vi "CRYPrefix Curve Name.vi"(0 "Type In":string="NameChange", 5 "Curves In":T2 {"Z data" items=["dB", "Lin"]; "X data" items=["dB", "Lin"]; "Y data" items=["dB", "Lin"]; "Z dB ref" format="%.1f"; "Z axis" items=["Log", "Lin"]; "X dB ref" format="%.1f"; "X axis" items=["Log", "Lin"]; "Y axis" items=["Log", "Lin"]; "Y dB ref" format="%.1f"; "Curve"."z" format="%.2f"; "Curve"."y" format="%.2f"; "Curve"."x" format="%.2f"}, 7 "Values In":T2 {"Z data" items=["dB", "Lin"]; "X data" items=["dB", "Lin"]; "Y data" items=["dB", "Lin"]; "Z dB ref" format="%.1f"; "Z axis" items=["Log", "Lin"]; "X dB ref" format="%.1f"; "X axis" items=["Log", "Lin"]; "Y axis" items=["Log", "Lin"]; "Y dB ref" format="%.1f"; "Curve"."z" format="%.2f"; "Curve"."y" format="%.2f"; "Curve"."x" format="%.2f"}, 9 "Results In":T4 {"Margin" format="%.2f"}, 11 "Waves In":T6 {"Y dB ref" format="%.1f"; "Y axis" items=["Log", "Lin"]; "Y data" items=["dB", "Lin"]; "X data" items=["dB", "Lin"]}, 12 "Repeat State Array In":T1(array[cluster])) -> (6 "Curves Out":T2 {"Z data" items=["dB", "Lin"]; "X data" items=["dB", "Lin"]; "Y data" items=["dB", "Lin"]; "Z dB ref" format="%.1f"; "Z axis" items=["Log", "Lin"]; "X dB ref" format="%.1f"; "X axis" items=["Log", "Lin"]; "Y axis" items=["Log", "Lin"]; "Y dB ref" format="%.1f"; "Curve"."z" format="%.2f"; "Curve"."y" format="%.2f"; "Curve"."x" format="%.2f"}, 8 "Values Out":T2 {"Z data" items=["dB", "Lin"]; "X data" items=["dB", "Lin"]; "Y data" items=["dB", "Lin"]; "Z dB ref" format="%.1f"; "Z axis" items=["Log", "Lin"]; "X dB ref" format="%.1f"; "X axis" items=["Log", "Lin"]; "Y axis" items=["Log", "Lin"]; "Y dB ref" format="%.1f"; "Curve"."z" format="%.2f"; "Curve"."y" format="%.2f"; "Curve"."x" format="%.2f"}, 10 "Results Out":T4 {"Margin" format="%.2f"}, 15 "Waves Out":T6 {"Y dB ref" format="%.1f"; "Y axis" items=["Log", "Lin"]; "Y data" items=["dB", "Lin"]; "X data" items=["dB", "Lin"]})   [LabVIEW 2013]
uses:
  Typedef Control/CRYData Cluster Array.ctl
  Typedef Control/CRYData Cluster.ctl
  Typedef Control/CRYResult Cluster Array.ctl
  Typedef Control/CRYResult Cluster.ctl
  Typedef Control/CRYWaveform Cluster Array.ctl
  Typedef Control/CRYWaveform Cluster.ctl
  CRYProject Run Control Global.vi
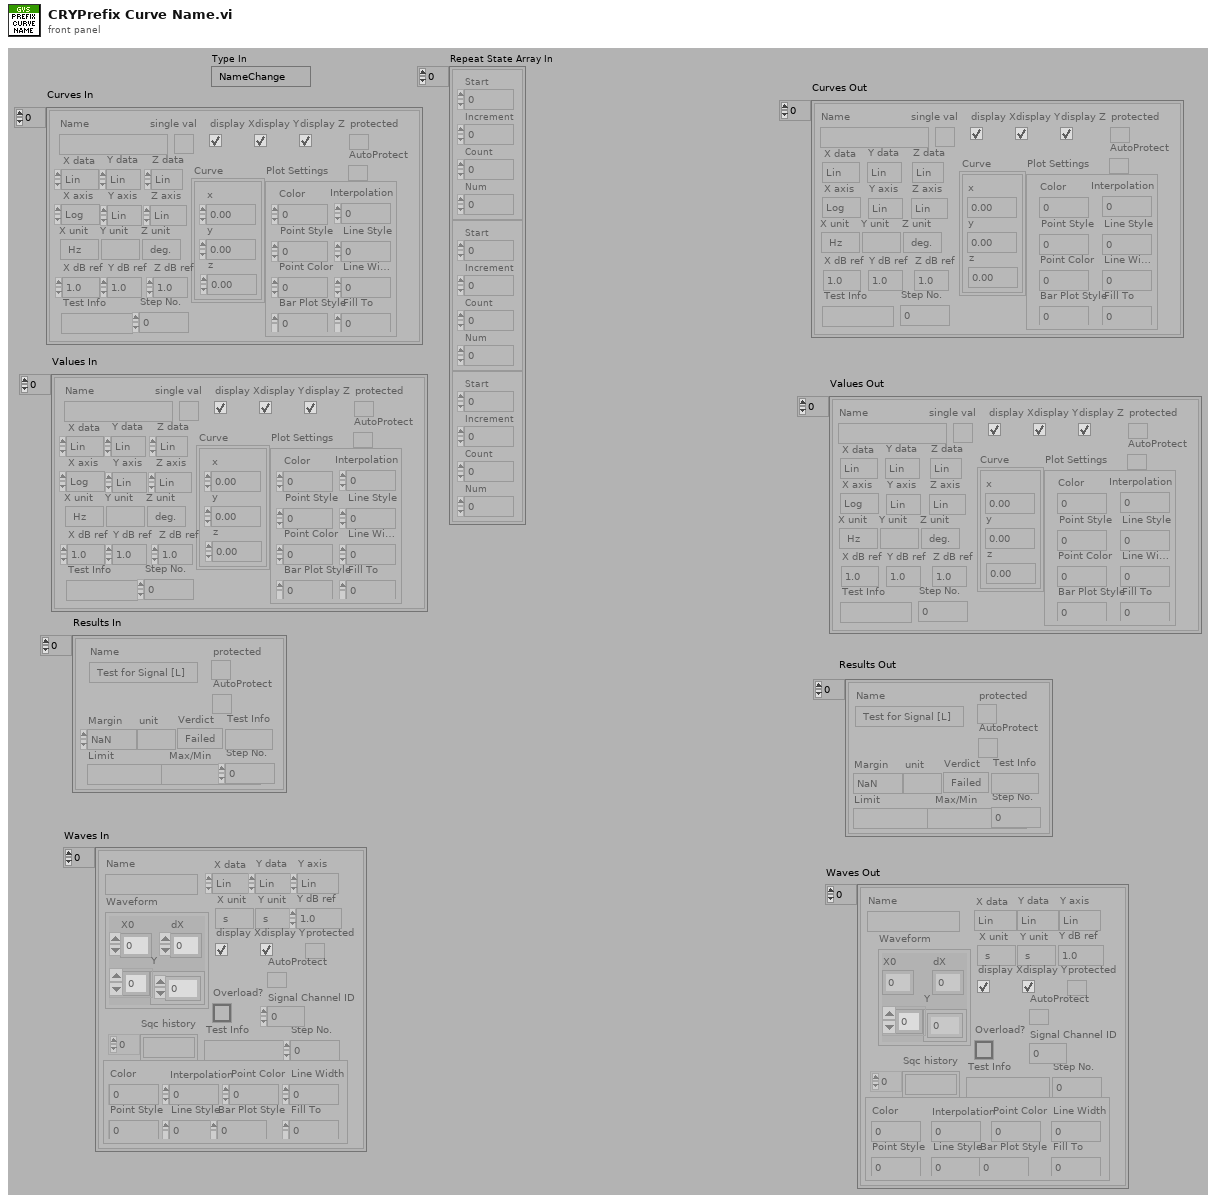
[diagram p1: front panel]
types:
  T1 = cluster{"Start":dbl, "Increment":dbl, "Count":i32, "Num":i32}[]
  T2 = typedef "CRYData Cluster Array.ctl" = T3[]
  T3 = typedef "CRYData Cluster.ctl" = cluster{"Name":string, "Curve":cluster{"x":dbl, "y":dbl, "z":dbl}[], "X data":u16, "Y data":u16, "Z data":u16, "X axis":u16, "Y axis":u16, "Z axis":u16, "X unit":string, "Y unit":string, "Z unit":string, "X dB ref":dbl, "Y dB ref":dbl, "Z dB ref":dbl, "single val":bool, "protected":bool, "display X":bool, "display Y":bool, "display Z":bool, "Test Info":string, "Step No.":i32, "Plot Settings":cluster{"Color":u32, "Interpolation":u8, "Point Style":u8, "Line Style":u8, "Point Color":u32, "Line Width":u8, "Bar Plot Style":u8, "Fill To":i16}, "AutoProtect":bool}
  T4 = typedef "CRYResult Cluster Array.ctl" = T5[]
  T5 = typedef "CRYResult Cluster.ctl" = cluster{"Name":string, "Margin":dbl, "unit":string, "Verdict":bool, "Limit":string, "Max/Min":string, "protected":bool, "Step No.":i32, "Test Info":string, "AutoProtect":bool}
  T6 = typedef "CRYWaveform Cluster Array.ctl" = T7[]
  T7 = typedef "CRYWaveform Cluster.ctl" = cluster{"Waveform":cluster{"X0":dbl, "dX":dbl, "Y":sgl[]}, "X data":u16, "Y data":u16, "Y axis":u16, "X unit":string, "Y unit":string, "Y dB ref":dbl, "display Y":bool, "display X":bool, "Overload?":bool, "Test Info":string, "Step No.":i32, "Name":string, "protected":bool, "Sqc history":string[], "Signal Channel ID":i32, "Plot Settings":cluster{"Color":u32, "Interpolation":u8, "Point Style":u8, "Line Style":u8, "Point Color":u32, "Line Width":u8, "Bar Plot Style":u8, "Fill To":i16}, "AutoProtect":bool}
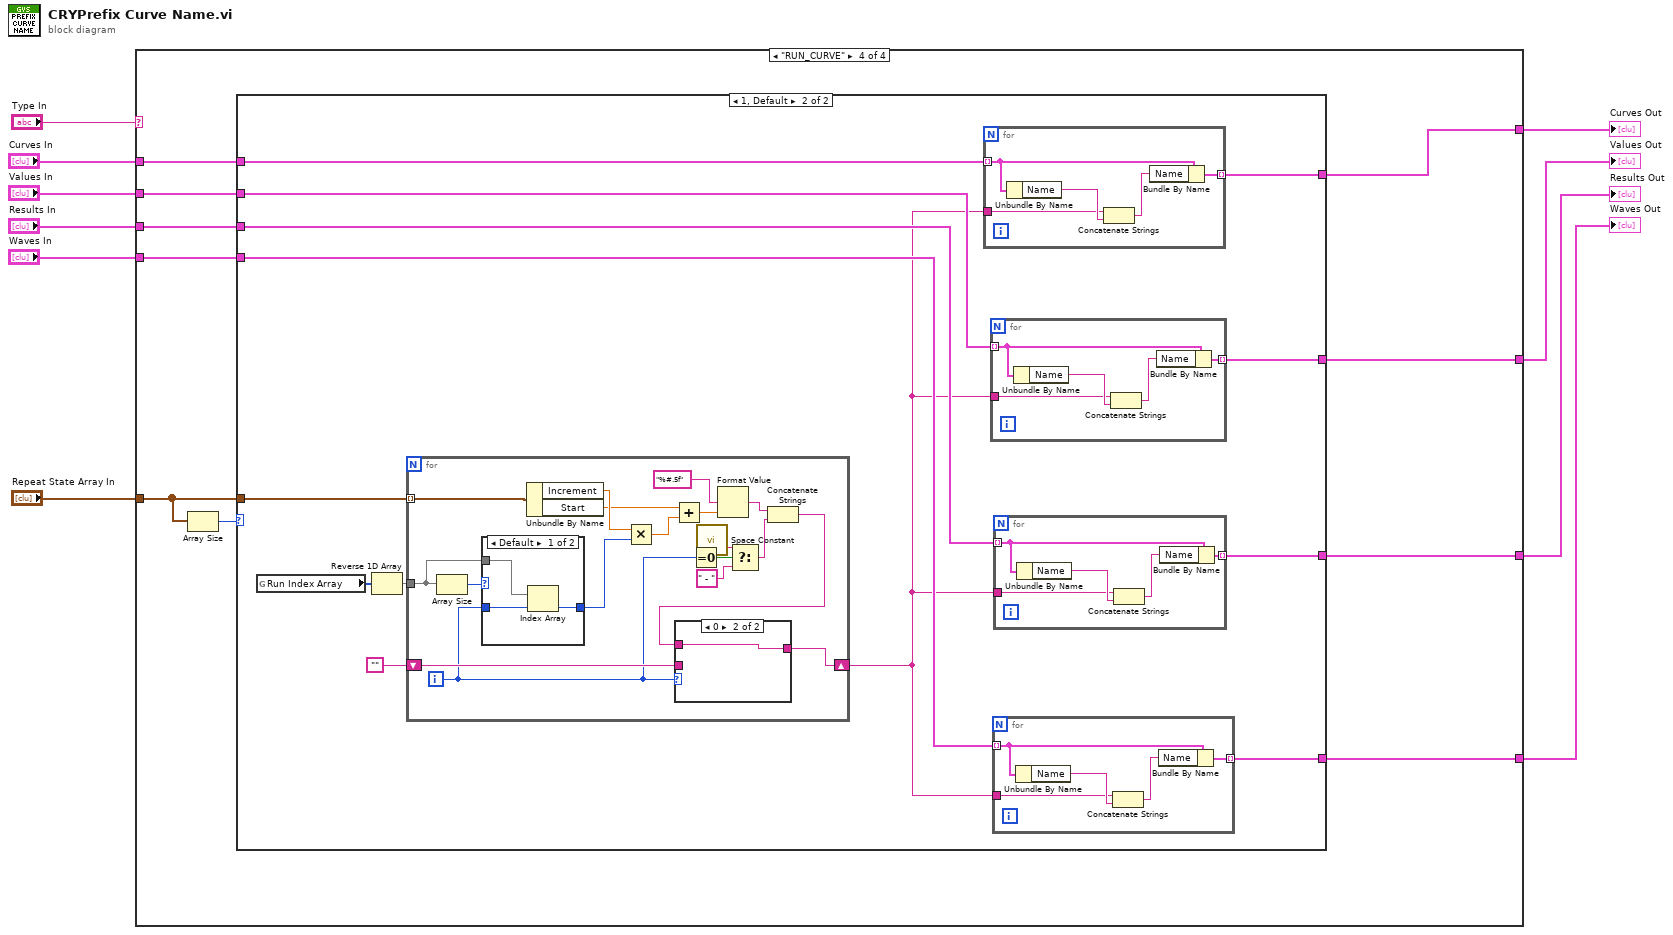
[diagram p0: block diagram]
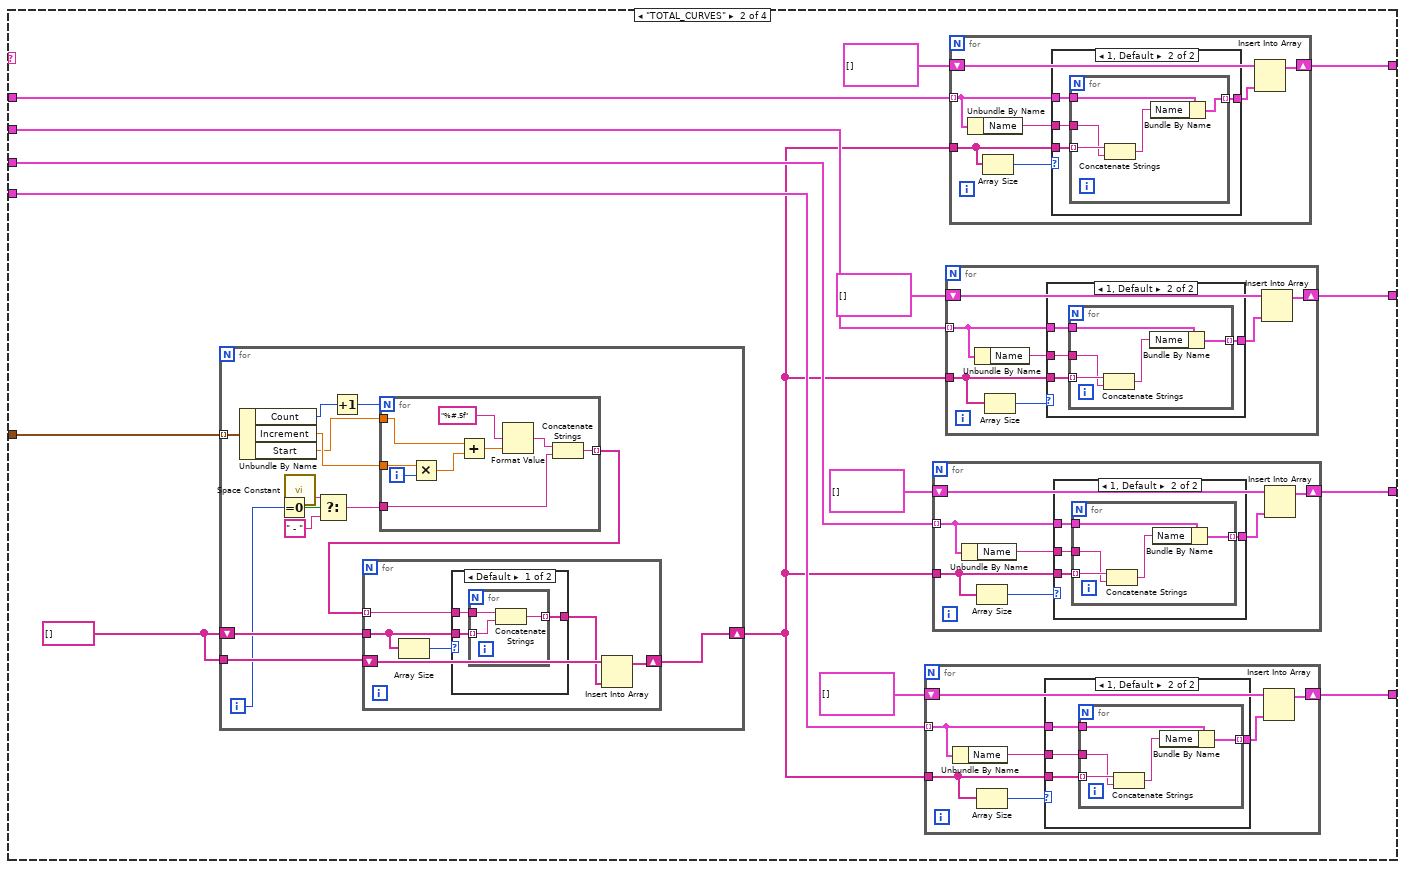
[diagram p3: hidden frame]
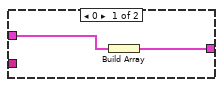
[diagram p4: hidden frame]
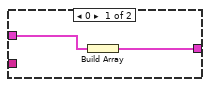
[diagram p5: hidden frame]
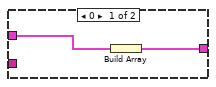
[diagram p6: hidden frame]
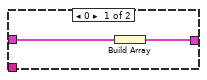
[diagram p7: hidden frame]
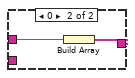
[diagram p8: hidden frame]
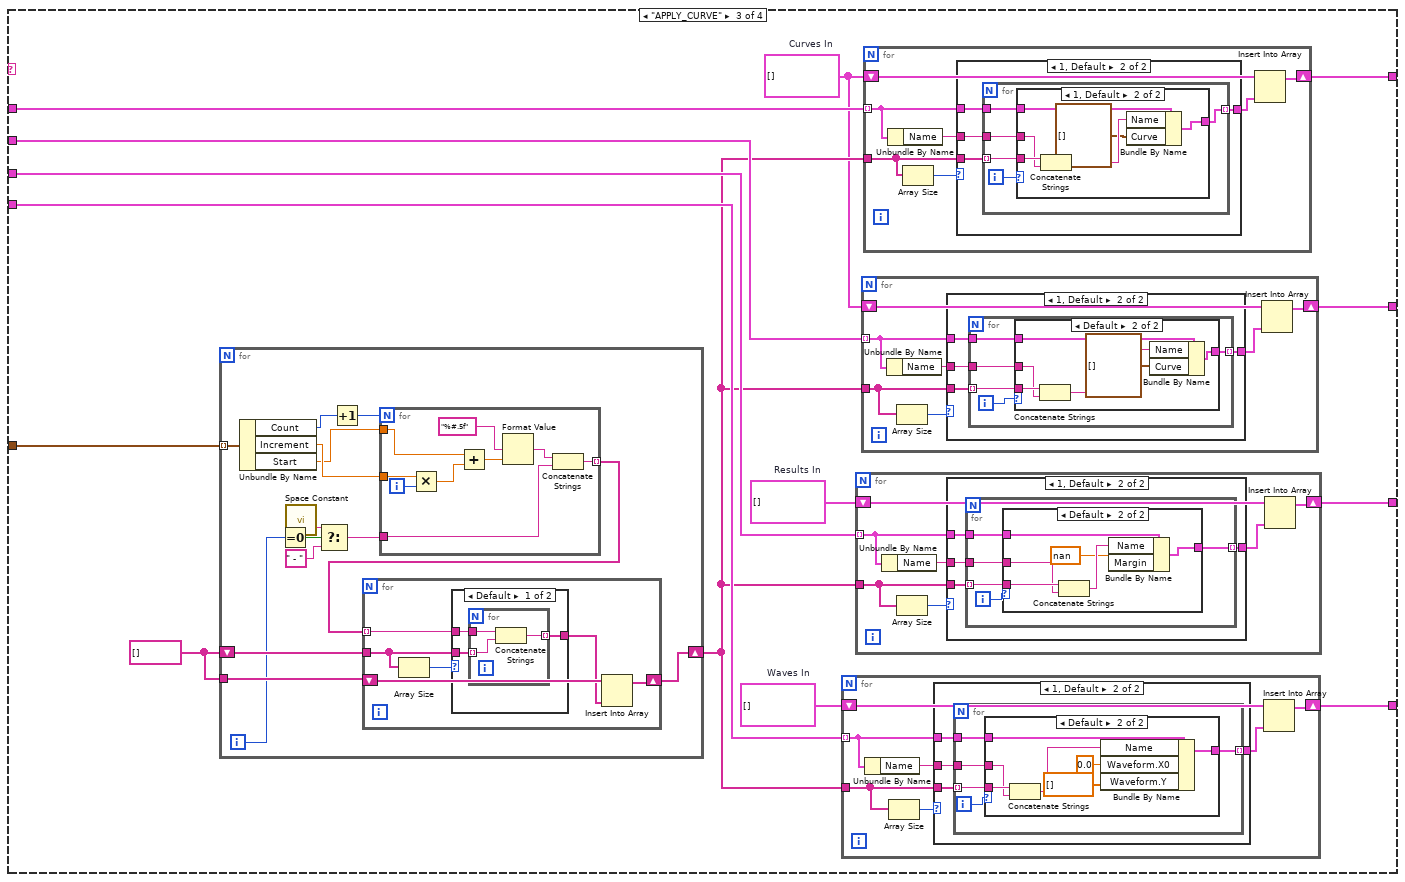
[diagram p9: hidden frame]
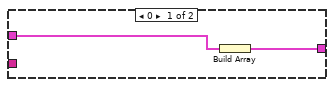
[diagram p10: hidden frame]
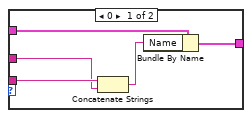
[diagram p11: hidden frame]
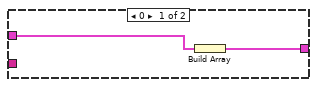
[diagram p12: hidden frame]
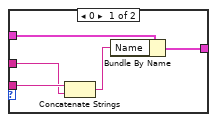
[diagram p13: hidden frame]
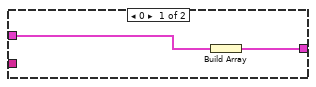
[diagram p14: hidden frame]
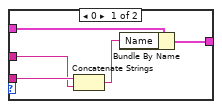
[diagram p15: hidden frame]
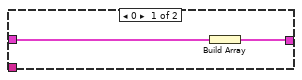
[diagram p16: hidden frame]
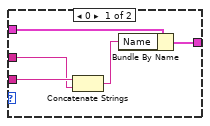
[diagram p17: hidden frame]
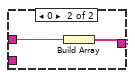
[diagram p18: hidden frame]
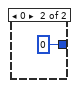
[diagram p20: hidden frame]
diagram:
  n1 = case shown="\"RUN_CURVE\"" "Type In" {
    tunnel: "Curves In" -> [_ w23 w146 w312]
    tunnel: "Repeat State Array In" -> [_ w24 w147 w308]
    tunnel: "Values In" -> [_ w22 w145 w311]
    tunnel: "Results In" -> [_ w20 w144 w310]
    tunnel: "Waves In" -> [_ w19 w143 w309]
    tunnel: [_ w15 w139 w307] -> w4
    tunnel: [_ w14 w138 w306] -> w3
    tunnel: [_ w13 w137 w305] -> w2
    tunnel: [_ w12 w136 w304] -> w1
    frame Default {
    }
    frame "TOTAL_CURVES" {
      w25 = string[] []
      n2 = for {
        tunnel: w24 -> [w111] mode=indexing
        shift-right: [w106] -> w18
        shift-left: w25 -> [w108]
        tunnel: w25 -> [w107]
        i -> [w99]
        n3 = Unbundle By Name(w111) -> ("Count"=w105:i32, "Increment"=w110:dbl, "Start"=w104:dbl)
        n4 = Equal To 0?(x=w99) -> (x = 0?=w102:bool)
        n5 = call <vilib>:"Space Constant.vi"() -> ("String"=w100:string)
        n6 = Select(t=w100, s=w102, f=" - " ("string")) -> (s? t:f=w98:string)
        n7 = Increment(x=w105) -> (x+1=w103:i32)
        n8 = for {
          N: w103 -> [_]
          tunnel: w104 -> [w134]
          tunnel: w110 -> [w133]
          tunnel: [w130] -> w109 mode=indexing
          tunnel: w98 -> [w126]
          i -> [w132]
          n9 = Multiply(x=w133, y=w132) -> (x*y=w131:dbl)
          n10 = Add(x=w134, y=w131) -> (x+y=w128:dbl)
          n11 = Format Value(format string="%#.5f", value (0)=w128) -> (output string=w127:string)  [unwired: 1 in]
          n12 = Concatenate Strings(w127, w126) -> (w130:string)
        }
        n13 = for {
          tunnel: w109 -> [w117] mode=indexing
          tunnel: w108 -> [w113]
          shift-right: [w115] -> w106
          shift-left: w107 -> [w116]
          n14 = Array Size(array=w113) -> (size(s)=w112:i32)
          n15 = case shown="Default" w112 {
            tunnel: w117 -> [w120 w125]
            tunnel: w113 -> [w119 _]
            tunnel: [w118 w124] -> w114
            frame Default {
              n16 = for {
                tunnel: w120 -> [w123]
                tunnel: w119 -> [w122] mode=indexing
                tunnel: [w121] -> w118 mode=indexing
                n17 = Concatenate Strings(w123, w122) -> (w121:string)
              }
            }
            frame 0 {
              n18 = Build Array(w125) -> (w124:string[])
            }
          }
          n19 = Insert Into Array(array=w116, new element=w114) -> (w115:string[])  [unwired: 1 in]
        }
      }
      n20 = for {
        tunnel: w19 -> [w31] mode=indexing
        tunnel: w18 -> [w27]
        shift-right: [w28] -> w12
        shift-left: T6 [] ("Waves In") -> [w30]
        n21 = Unbundle By Name(w31) -> ("Name"=w32:string)
        n22 = Array Size(array=w27) -> (size(s)=w26:i32)
        n23 = case shown="1, Default" w26 {
          tunnel: w32 -> [_ w38]
          tunnel: w31 -> [w34 w37]
          tunnel: [w33 w36] -> w29
          tunnel: w27 -> [_ w35]
          frame 0 {
            n24 = Build Array(w34) -> (w33:T7[])
          }
          frame 1, Default {
            n25 = for {
              tunnel: w38 -> [w42]
              tunnel: w35 -> [w43] mode=indexing
              tunnel: w37 -> [w41]
              tunnel: [w39] -> w36 mode=indexing
              n26 = Concatenate Strings(w43, w42) -> (w40:string)
              n27 = Bundle By Name(cluster=w41, "Name"=w40) -> (w39:T7)
            }
          }
        }
        n28 = Insert Into Array(array=w30, new element=w29) -> (w28:T6)  [unwired: 1 in]
      }
      n29 = for {
        tunnel: w20 -> [w49] mode=indexing
        tunnel: w18 -> [w45]
        shift-right: [w46] -> w13
        shift-left: T4 [] ("Results In") -> [w48]
        n30 = Unbundle By Name(w49) -> ("Name"=w50:string)
        n31 = Array Size(array=w45) -> (size(s)=w44:i32)
        n32 = case shown="1, Default" w44 {
          tunnel: w50 -> [_ w56]
          tunnel: w45 -> [_ w55]
          tunnel: w49 -> [w52 w54]
          tunnel: [w51 w53] -> w47
          frame 0 {
            n33 = Build Array(w52) -> (w51:T5[])
          }
          frame 1, Default {
            n34 = for {
              tunnel: w56 -> [w60]
              tunnel: w55 -> [w61] mode=indexing
              tunnel: w54 -> [w59]
              tunnel: [w57] -> w53 mode=indexing
              n35 = Concatenate Strings(w61, w60) -> (w58:string)
              n36 = Bundle By Name(cluster=w59, "Name"=w58) -> (w57:T5)
            }
          }
        }
        n37 = Insert Into Array(array=w48, new element=w47) -> (w46:T4)  [unwired: 1 in]
      }
      n38 = for {
        tunnel: w22 -> [w67] mode=indexing
        tunnel: w18 -> [w63]
        shift-right: [w64] -> w14
        shift-left: T2 [] ("Values In") -> [w66]
        n39 = Unbundle By Name(w67) -> ("Name"=w68:string)
        n40 = Array Size(array=w63) -> (size(s)=w62:i32)
        n41 = case shown="1, Default" w62 {
          tunnel: w68 -> [_ w74]
          tunnel: w67 -> [w70 w73]
          tunnel: [w69 w72] -> w65
          tunnel: w63 -> [_ w71]
          frame 0 {
            n42 = Build Array(w70) -> (w69:T3[])
          }
          frame 1, Default {
            n43 = for {
              tunnel: w74 -> [w78]
              tunnel: w71 -> [w79] mode=indexing
              tunnel: w73 -> [w77]
              tunnel: [w75] -> w72 mode=indexing
              n44 = Concatenate Strings(w79, w78) -> (w76:string)
              n45 = Bundle By Name(cluster=w77, "Name"=w76) -> (w75:T3)
            }
          }
        }
        n46 = Insert Into Array(array=w66, new element=w65) -> (w64:T2)  [unwired: 1 in]
      }
      n47 = for {
        tunnel: w23 -> [w85] mode=indexing
        tunnel: w18 -> [w81]
        shift-right: [w82] -> w15
        shift-left: T2 [] ("Curves In") -> [w84]
        n48 = Unbundle By Name(w85) -> ("Name"=w86:string)
        n49 = Array Size(array=w81) -> (size(s)=w80:i32)
        n50 = case shown="1, Default" w80 {
          tunnel: w86 -> [_ w92]
          tunnel: w81 -> [_ w91]
          tunnel: w85 -> [w88 w90]
          tunnel: [w87 w89] -> w83
          frame 0 {
            n51 = Build Array(w88) -> (w87:T3[])
          }
          frame 1, Default {
            n52 = for {
              tunnel: w92 -> [w96]
              tunnel: w91 -> [w97] mode=indexing
              tunnel: w90 -> [w95]
              tunnel: [w93] -> w89 mode=indexing
              n53 = Concatenate Strings(w97, w96) -> (w94:string)
              n54 = Bundle By Name(cluster=w95, "Name"=w94) -> (w93:T3)
            }
          }
        }
        n55 = Insert Into Array(array=w84, new element=w83) -> (w82:T2)  [unwired: 1 in]
      }
    }
    frame "APPLY_CURVE" {
      w140 = T4 []  # Results In
      w141 = T6 []  # Waves In
      w135 = T2 []  # Curves In
      w148 = string[] []
      n56 = for {
        tunnel: w147 -> [w279] mode=indexing
        shift-right: [w274] -> w142
        shift-left: w148 -> [w276]
        tunnel: w148 -> [w275]
        i -> [w267]
        n57 = Unbundle By Name(w279) -> ("Count"=w273:i32, "Increment"=w278:dbl, "Start"=w272:dbl)
        n58 = Equal To 0?(x=w267) -> (x = 0?=w270:bool)
        n59 = call <vilib>:"Space Constant.vi"() -> ("String"=w269:string)
        n60 = Select(t=w269, s=w270, f=" - " ("string")) -> (s? t:f=w266:string)
        n61 = Increment(x=w273) -> (x+1=w271:i32)
        n62 = for {
          N: w271 -> [_]
          tunnel: w272 -> [w302]
          tunnel: w278 -> [w301]
          tunnel: [w298] -> w277 mode=indexing
          tunnel: w266 -> [w294]
          i -> [w300]
          n63 = Multiply(x=w301, y=w300) -> (x*y=w299:dbl)
          n64 = Add(x=w302, y=w299) -> (x+y=w296:dbl)
          n65 = Format Value(format string="%#.5f", value (0)=w296) -> (output string=w295:string)  [unwired: 1 in]
          n66 = Concatenate Strings(w295, w294) -> (w298:string)
        }
        n67 = for {
          tunnel: w277 -> [w285] mode=indexing
          tunnel: w276 -> [w281]
          shift-right: [w283] -> w274
          shift-left: w275 -> [w284]
          n68 = Array Size(array=w281) -> (size(s)=w280:i32)
          n69 = case shown="Default" w280 {
            tunnel: w285 -> [w288 w293]
            tunnel: w281 -> [w287 _]
            tunnel: [w286 w292] -> w282
            frame Default {
              n70 = for {
                tunnel: w288 -> [w291]
                tunnel: w287 -> [w290] mode=indexing
                tunnel: [w289] -> w286 mode=indexing
                n71 = Concatenate Strings(w291, w290) -> (w289:string)
              }
            }
            frame 0 {
              n72 = Build Array(w293) -> (w292:string[])
            }
          }
          n73 = Insert Into Array(array=w284, new element=w282) -> (w283:string[])  [unwired: 1 in]
        }
      }
      n74 = for {
        tunnel: w143 -> [w154] mode=indexing
        tunnel: w142 -> [w150]
        shift-right: [w151] -> w136
        shift-left: w141 -> [w153]
        n75 = Unbundle By Name(w154) -> ("Name"=w155:string)
        n76 = Array Size(array=w150) -> (size(s)=w149:i32)
        n77 = case shown="1, Default" w149 {
          tunnel: w155 -> [_ w161]
          tunnel: w154 -> [w157 w160]
          tunnel: [w156 w159] -> w152
          tunnel: w150 -> [_ w158]
          frame 0 {
            n78 = Build Array(w157) -> (w156:T7[])
          }
          frame 1, Default {
            n79 = for {
              tunnel: w161 -> [w165]
              tunnel: w158 -> [w166] mode=indexing
              tunnel: w160 -> [w164]
              tunnel: [w163] -> w159 mode=indexing
              i -> [w162]
              n80 = case shown="Default" w162 {
                tunnel: w166 -> [w171 w178]
                tunnel: w165 -> [w170 w177]
                tunnel: w164 -> [w169 w176]
                tunnel: [w167 w174] -> w163
                frame 0 {
                  n81 = Concatenate Strings(w171, w170) -> (w168:string)
                  n82 = Bundle By Name(cluster=w169, "Name"=w168) -> (w167:T7)
                }
                frame Default {
                  n83 = Concatenate Strings(w178, w177) -> (w175:string)
                  n84 = Bundle By Name(cluster=w176, "Name"=w175, "Waveform.X0"=0.0, "Waveform.Y"=sgl[] []) -> (w174:T7)
                }
              }
            }
          }
        }
        n85 = Insert Into Array(array=w153, new element=w152) -> (w151:T6)  [unwired: 1 in]
      }
      n86 = for {
        tunnel: w144 -> [w184] mode=indexing
        tunnel: w142 -> [w180]
        shift-right: [w181] -> w137
        shift-left: w140 -> [w183]
        n87 = Unbundle By Name(w184) -> ("Name"=w185:string)
        n88 = Array Size(array=w180) -> (size(s)=w179:i32)
        n89 = case shown="1, Default" w179 {
          tunnel: w185 -> [_ w191]
          tunnel: w180 -> [_ w190]
          tunnel: w184 -> [w187 w189]
          tunnel: [w186 w188] -> w182
          frame 0 {
            n90 = Build Array(w187) -> (w186:T5[])
          }
          frame 1, Default {
            n91 = for {
              tunnel: w191 -> [w195]
              tunnel: w190 -> [w196] mode=indexing
              tunnel: w189 -> [w194]
              tunnel: [w193] -> w188 mode=indexing
              i -> [w192]
              n92 = case shown="Default" w192 {
                tunnel: w196 -> [w201 w207]
                tunnel: w195 -> [w200 w206]
                tunnel: w194 -> [w199 w205]
                tunnel: [w197 w203] -> w193
                frame 0 {
                  n93 = Concatenate Strings(w201, w200) -> (w198:string)
                  n94 = Bundle By Name(cluster=w199, "Name"=w198) -> (w197:T5)
                }
                frame Default {
                  n95 = Concatenate Strings(w207, w206) -> (w204:string)
                  n96 = Bundle By Name(cluster=w205, "Name"=w204, "Margin"=nan) -> (w203:T5)
                }
              }
            }
          }
        }
        n97 = Insert Into Array(array=w183, new element=w182) -> (w181:T4)  [unwired: 1 in]
      }
      n98 = for {
        tunnel: w145 -> [w213] mode=indexing
        tunnel: w142 -> [w209]
        shift-right: [w210] -> w138
        shift-left: w135 -> [w212]
        n99 = Unbundle By Name(w213) -> ("Name"=w214:string)
        n100 = Array Size(array=w209) -> (size(s)=w208:i32)
        n101 = case shown="1, Default" w208 {
          tunnel: w214 -> [_ w220]
          tunnel: w213 -> [w216 w219]
          tunnel: [w215 w218] -> w211
          tunnel: w209 -> [_ w217]
          frame 0 {
            n102 = Build Array(w216) -> (w215:T3[])
          }
          frame 1, Default {
            n103 = for {
              tunnel: w220 -> [w224]
              tunnel: w217 -> [w225] mode=indexing
              tunnel: w219 -> [w223]
              tunnel: [w222] -> w218 mode=indexing
              i -> [w221]
              n104 = case shown="Default" w221 {
                tunnel: w225 -> [w230 w236]
                tunnel: w224 -> [w229 w235]
                tunnel: w223 -> [w228 w234]
                tunnel: [w226 w232] -> w222
                frame 0 {
                  n105 = Concatenate Strings(w230, w229) -> (w227:string)
                  n106 = Bundle By Name(cluster=w228, "Name"=w227) -> (w226:T3)
                }
                frame Default {
                  n107 = Concatenate Strings(w236, w235) -> (w233:string)
                  n108 = Bundle By Name(cluster=w234, "Name"=w233, "Curve"=cluster{"x":dbl, "y":dbl, "z":dbl}[] []) -> (w232:T3)
                }
              }
            }
          }
        }
        n109 = Insert Into Array(array=w212, new element=w211) -> (w210:T2)  [unwired: 1 in]
      }
      n110 = for {
        tunnel: w146 -> [w242] mode=indexing
        tunnel: w142 -> [w238]
        shift-right: [w239] -> w139
        shift-left: w135 -> [w241]
        n111 = Unbundle By Name(w242) -> ("Name"=w243:string)
        n112 = Array Size(array=w238) -> (size(s)=w237:i32)
        n113 = case shown="1, Default" w237 {
          tunnel: w243 -> [_ w249]
          tunnel: w238 -> [_ w248]
          tunnel: w242 -> [w245 w247]
          tunnel: [w244 w246] -> w240
          frame 0 {
            n114 = Build Array(w245) -> (w244:T3[])
          }
          frame 1, Default {
            n115 = for {
              tunnel: w249 -> [w253]
              tunnel: w248 -> [w254] mode=indexing
              tunnel: w247 -> [w252]
              tunnel: [w251] -> w246 mode=indexing
              i -> [w250]
              n116 = case shown="1, Default" w250 {
                tunnel: w254 -> [w259 w265]
                tunnel: w253 -> [w258 w264]
                tunnel: w252 -> [w257 w263]
                tunnel: [w255 w261] -> w251
                frame 0 {
                  n117 = Concatenate Strings(w259, w258) -> (w256:string)
                  n118 = Bundle By Name(cluster=w257, "Name"=w256) -> (w255:T3)
                }
                frame 1, Default {
                  n119 = Concatenate Strings(w265, w264) -> (w262:string)
                  n120 = Bundle By Name(cluster=w263, "Name"=w262, "Curve"=cluster{"x":dbl, "y":dbl, "z":dbl}[] []) -> (w261:T3)
                }
              }
            }
          }
        }
        n121 = Insert Into Array(array=w241, new element=w240) -> (w239:T2)  [unwired: 1 in]
      }
    }
    frame "RUN_CURVE" {
      n122 = Array Size(array=w308) -> (size(s)=w303:i32)
      n123 = case shown="1, Default" w303 {
        tunnel: w312 -> [w316 w329]
        tunnel: w311 -> [w315 w328]
        tunnel: w310 -> [w314 w327]
        tunnel: w309 -> [w313 w326]
        tunnel: w308 -> [_ w324]
        tunnel: [w316 w322] -> w307
        tunnel: [w315 w321] -> w306
        tunnel: [w314 w320] -> w305
        tunnel: [w313 w319] -> w304
        frame 0 {
        }
        frame 1, Default {
          n124 = global read "CRYProject Run Control Global.vi" "Run Index Array"() -> (w323:u32[])
          n125 = Reverse 1D Array(array=w323) -> (reversed array=w317:u32[])
          n126 = for {
            tunnel: w324 -> [w347] mode=indexing
            shift-right: [w338] -> w325
            shift-left: "" -> [w344]
            tunnel: w317 -> [w336]
            i -> [w331]
            n127 = Array Size(array=w336) -> (size(s)=w337:i32)
            n128 = case shown="Default" w337 {
              tunnel: w336 -> [w350 _]
              tunnel: w331 -> [w349 _]
              tunnel: [w348 u32 0 ("Numeric")] -> w335
              frame Default {
                n129 = Index Array(array=w350, index=w349) -> (element=w348:u32)
              }
              frame 0 {
              }
            }
            n130 = Unbundle By Name(w347) -> ("Increment"=w346:dbl, "Start"=w343:dbl)
            n131 = Multiply(x=w346, y=w335) -> (x*y=w342:dbl)
            n132 = Add(x=w343, y=w342) -> (x+y=w340:dbl)
            n133 = Equal To 0?(x=w331) -> (x = 0?=w334:bool)
            n134 = call <vilib>:"Space Constant.vi"() -> ("String"=w330:string)
            n135 = Format Value(format string="%#.5f", value (0)=w340) -> (output string=w339:string)  [unwired: 1 in]
            n136 = Select(t=w330, s=w334, f=" - " ("string")) -> (s? t:f=w332:string)
            n137 = Concatenate Strings(w339, w332) -> (w345:string)
            n138 = case shown="0" w331 {
              tunnel: w345 -> [w354 w355]
              tunnel: w344 -> [w353 _]
              tunnel: [w352 w355] -> w338
              frame Default {
                n139 = Concatenate Strings(w354, w353) -> (w352:string)
              }
              frame 0 {
              }
            }
          }
          n140 = for {
            tunnel: w329 -> [w373] mode=indexing
            tunnel: w325 -> [w374]
            tunnel: [w371] -> w322 mode=indexing
            n141 = Unbundle By Name(w373) -> ("Name"=w375:string)
            n142 = Concatenate Strings(w374, w375) -> (w372:string)
            n143 = Bundle By Name(cluster=w373, "Name"=w372) -> (w371:T3)
          }
          n144 = for {
            tunnel: w328 -> [w368] mode=indexing
            tunnel: w325 -> [w369]
            tunnel: [w366] -> w321 mode=indexing
            n145 = Unbundle By Name(w368) -> ("Name"=w370:string)
            n146 = Concatenate Strings(w369, w370) -> (w367:string)
            n147 = Bundle By Name(cluster=w368, "Name"=w367) -> (w366:T3)
          }
          n148 = for {
            tunnel: w326 -> [w358] mode=indexing
            tunnel: w325 -> [w359]
            tunnel: [w356] -> w319 mode=indexing
            n149 = Unbundle By Name(w358) -> ("Name"=w360:string)
            n150 = Concatenate Strings(w359, w360) -> (w357:string)
            n151 = Bundle By Name(cluster=w358, "Name"=w357) -> (w356:T7)
          }
          n152 = for {
            tunnel: w327 -> [w363] mode=indexing
            tunnel: w325 -> [w364]
            tunnel: [w361] -> w320 mode=indexing
            n153 = Unbundle By Name(w363) -> ("Name"=w365:string)
            n154 = Concatenate Strings(w364, w365) -> (w362:string)
            n155 = Bundle By Name(cluster=w363, "Name"=w362) -> (w361:T5)
          }
        }
      }
    }
  }
  "Curves Out" <- w4
  "Results Out" <- w2
  "Values Out" <- w3
  "Waves Out" <- w1
